vi "Build_Asylum_ReadString.vi"(8 "error in (no error)":errorcluster, 11 "parameterName":string) -> (0 "error out":errorcluster, 3 "String":string)   [LabVIEW 2016]
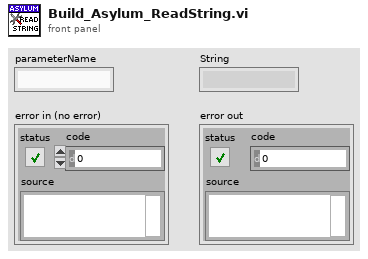
[diagram p1: front panel]
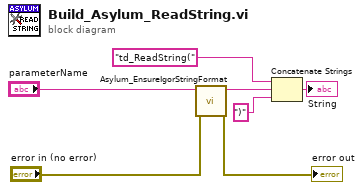
[diagram p0: block diagram]
diagram:
  n1 = call "Asylum_EnsureIgorStringFormat.vi"("error in (no error)"="error in (no error)", "Value"="parameterName") -> ("error out"=→"error out":errorcluster, "Value"=w4:string)  [unwired: 8 in]
  n2 = Concatenate Strings("td_ReadString(" ("string"), w4, ")" ("string")) -> (→"String":string)
